vi "Do.vi"(8 "error in":errorcluster, 10 "Actor in":refnum<class "Actor.lvclass">, 11 "Start Tau Write MSG":refnum<class "Start Tau Write MSG.lvclass">) -> (0 "error out":errorcluster, 2 "Actor out":refnum<class "Actor.lvclass">)   [LabVIEW 2014, in "Controller.lvlib" / "Start Tau Write MSG.lvclass"]
doc: "(<B>Filename</B>: Actor Framework.lvlib:Message.lvclass:Do.vi)\n\nDefines what a message does when it is received by an actor. Generally, a message instructs an actor to invoke one of its methods. By default, this method does nothing. A child class must override it to define behavior. Create a child class by using the Actor Framework Message Maker dialog box."
uses:
  Start Tau Write MSG.lvclass
  <vilib>/ActorFramework/Actor/Actor.lvclass
  Controller.lvclass
  Controller.lvclass/Controller.ctl
  File Actor/File Actor.lvclass
  Execute Write Taus/Exe Write Taus.lvclass
  Instr Exe Write to File/Instr Exe Write to File.lvclass/Instr Exe Write to File.ctl
  SuperActor/Ex Nested.lvclass/Ex Nested.ctl
  File Actor/File Actor.lvclass/File Actor.ctl
  <vilib>/ActorFramework/Actor/Actor.lvclass/Actor.ctl
  <vilib>/ActorFramework/Message Enqueuer/Message Enqueuer.lvclass/Message Enqueuer.ctl
  SuperActor/Write ID.vi
  File Actor/Write Cfg Header.vi
  File Actor/Write Exe Write.vi
  File Actor/Write Wait on Registration_.vi
  File Actor/Write Registration Complete.vi
  Instr Exe Write to File/Write MAP DVR.vi
  Instr Exe Write to File/Write DataObj.vi
  Accessors/Read Data Map.vi
  <vilib>/ActorFramework/Actor/Read Self Enqueuer.vi
  <vilib>/ActorFramework/Message Enqueuer/Enqueue.vi
  <vilib>/ActorFramework/Message Enqueuer/Init from Existing Queue.vi
  <vilib>/ActorFramework/Message Priority Queue/Priority Enqueue.vi
  <vilib>/ActorFramework/Message Enqueuer/Message Enqueuer.lvclass
  File Actor/Messages/To/Change File MSG/Change File MSG.lvclass
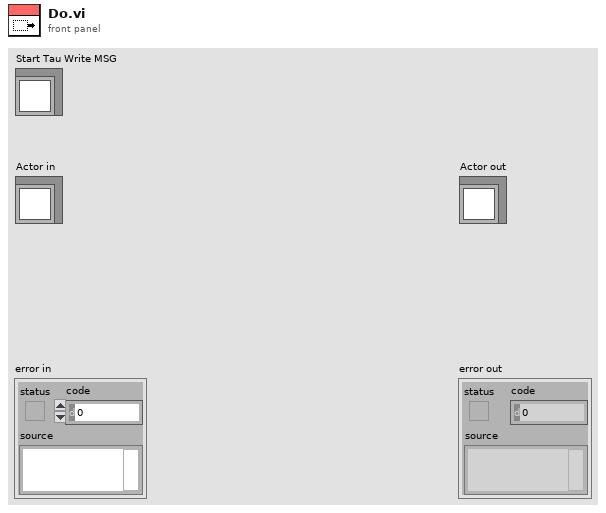
[diagram p1: front panel]
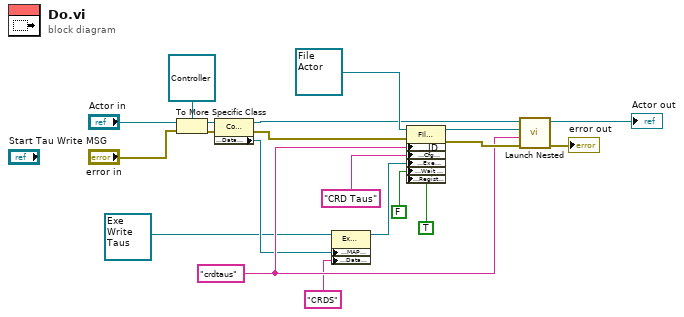
[diagram p0: block diagram]
diagram:
  w16 = "crdtaus" ("ID")
  n1 = To More Specific Class(target class=refnum<class "Controller.lvclass"> refnum ("Controller:Controller"), reference="Actor in", error in="error in") -> (specific class reference=w14:refnum<class "Controller.lvclass">, error out=w13:errorcluster)
  n2 = property class="Controller"(reference=w14, error in=w13) -> (reference out=w12:refnum<class "Controller.lvclass">, error out=w11:errorcluster, "Accessors:Data Map"=w10:refnum<data-value>)
  n3 = property class="Exe Write Taus"(reference=refnum<class "Exe Write Taus.lvclass"> refnum ("Controller:Exe Write Taus"), "Accessors:MAP DVR"=w10, "Accessors:DataObj"="CRDS" ("DataObj")) -> (reference out=w9:refnum<class "Exe Write Taus.lvclass">)  [unwired: 1 in, 1 out]
  n4 = property class="File Actor"(reference=refnum<class "File Actor.lvclass"> refnum ("File Library.lvlib:File Actor"), error in=w11, "Accessors:ID"=w16, "Accessors:Cfg Header"="CRD Taus" ("Cfg Header"), "Accessors:Exe Write"=w9, "Accessors:Wait on Registration_"=FALSE ("Wait on Registration_"), "Accessors:Registration Complete"=TRUE ("Registration Complete")) -> (reference out=w19:refnum<class "File Actor.lvclass">, error out=w18:errorcluster)
  n5 = call "Launch Nested.vi"("Error In"=w18, "ID"=w16, "Nested Actor"=w19, "Controller in"=w12) -> ("Error Out"=→"error out":errorcluster, "Controller out"=→"Actor out":refnum<class "Controller.lvclass">)  [unwired: 5 in, 1 out]
